vi "UHR-Fleezers Control (host) - 12.1.vi"() -> ()   [LabVIEW 2012] (continued)
  in  "Limits Enable":bool=TRUE caption="Enable"
  out "AI labels":string[](array[string])=["T1 Y", "T1 X", "T1 Sum", "T2 Y", "T2 X", "T2 Sum", "T1 FB X", "T1 FB Sum", "T2 FB X", "T2 FB Sum", "PSD Y", "PSD X", "PSD Y Sum"]
  in  "Save Trap Pos. Data":bool=TRUE
  in  "Lower Ch. Cap.":bool
  in  "Top 3 Harvard Syringe Pump Serial Port":refnum<visa-resource-name>="Top3Harvard"
  # "After"
  # "During"
  # "Trap On?"
  # "BD Flow ON?"
  # "Samp Flow ON?"
  # "Trap Trig. Fl.?"
  # "Zero It"
  # "Floor it\n(e.g., hp unwinding)"
  # "1"
  # "2"
  # "Fl. Down"
  # "Fl. Up"
  # "Bead sep"
  # "Trap Display:"
  # "APD Display:"
  # "DAQ"
  # "Trap Manipulation"
  # "Data Saving"
  # "Bead Calibration"
  # "Bottom Pump (#1)"
  # "Central Sample Channels"
  # "Top Pump (#3)"
  # "Rate param is ul/h\nVolume param is ul"
  # "Chemyx Pump 2"
  # "Units: \n1 = ml/m\n2 = ml/h\n3 = ul/m\n4 = ul/h"
  # "X"
  # "Amp switch 1st is disabled in the fpga"
  # "Y"
  # "Oscillate Set 1 freq. (debugging)"
  # "BD 1"
  # "BD 2"
  # "AOD Raster Scan"
  # "Approx. trap separations"
  # "X"
  # "Y"
  # "FPGA\nreading"
  # "DMA\ntransfer"
  # "APD Gates"
  # "APD 2"
  # "APD 1"
  # "X"
  # "2D"
  # "Y"
  # "1D"
  # "Green Laser Interlacing"
  # "Green FB Measurement"
  # "Digital Gate"
  # "Current Analog Control"
  # "Total AI Rates (NOT rates/trap)"
  # "(Samples/trap x Trap Sets)"
  # "(Samples/channel x\n8 if averaging (8 channels)\n4 if no averaging)"
  # "Trap 1"
  # "Trap 2"
  # "Flour./Trap 3"
  # "External Video Window"
  # "MCL Position Debugging"
  # "Temporary Control Storage\n(these used to be somewhere else, still want to keep them)"
  # "Y"
  # "X"
  # "Trap Position Difference Limits"
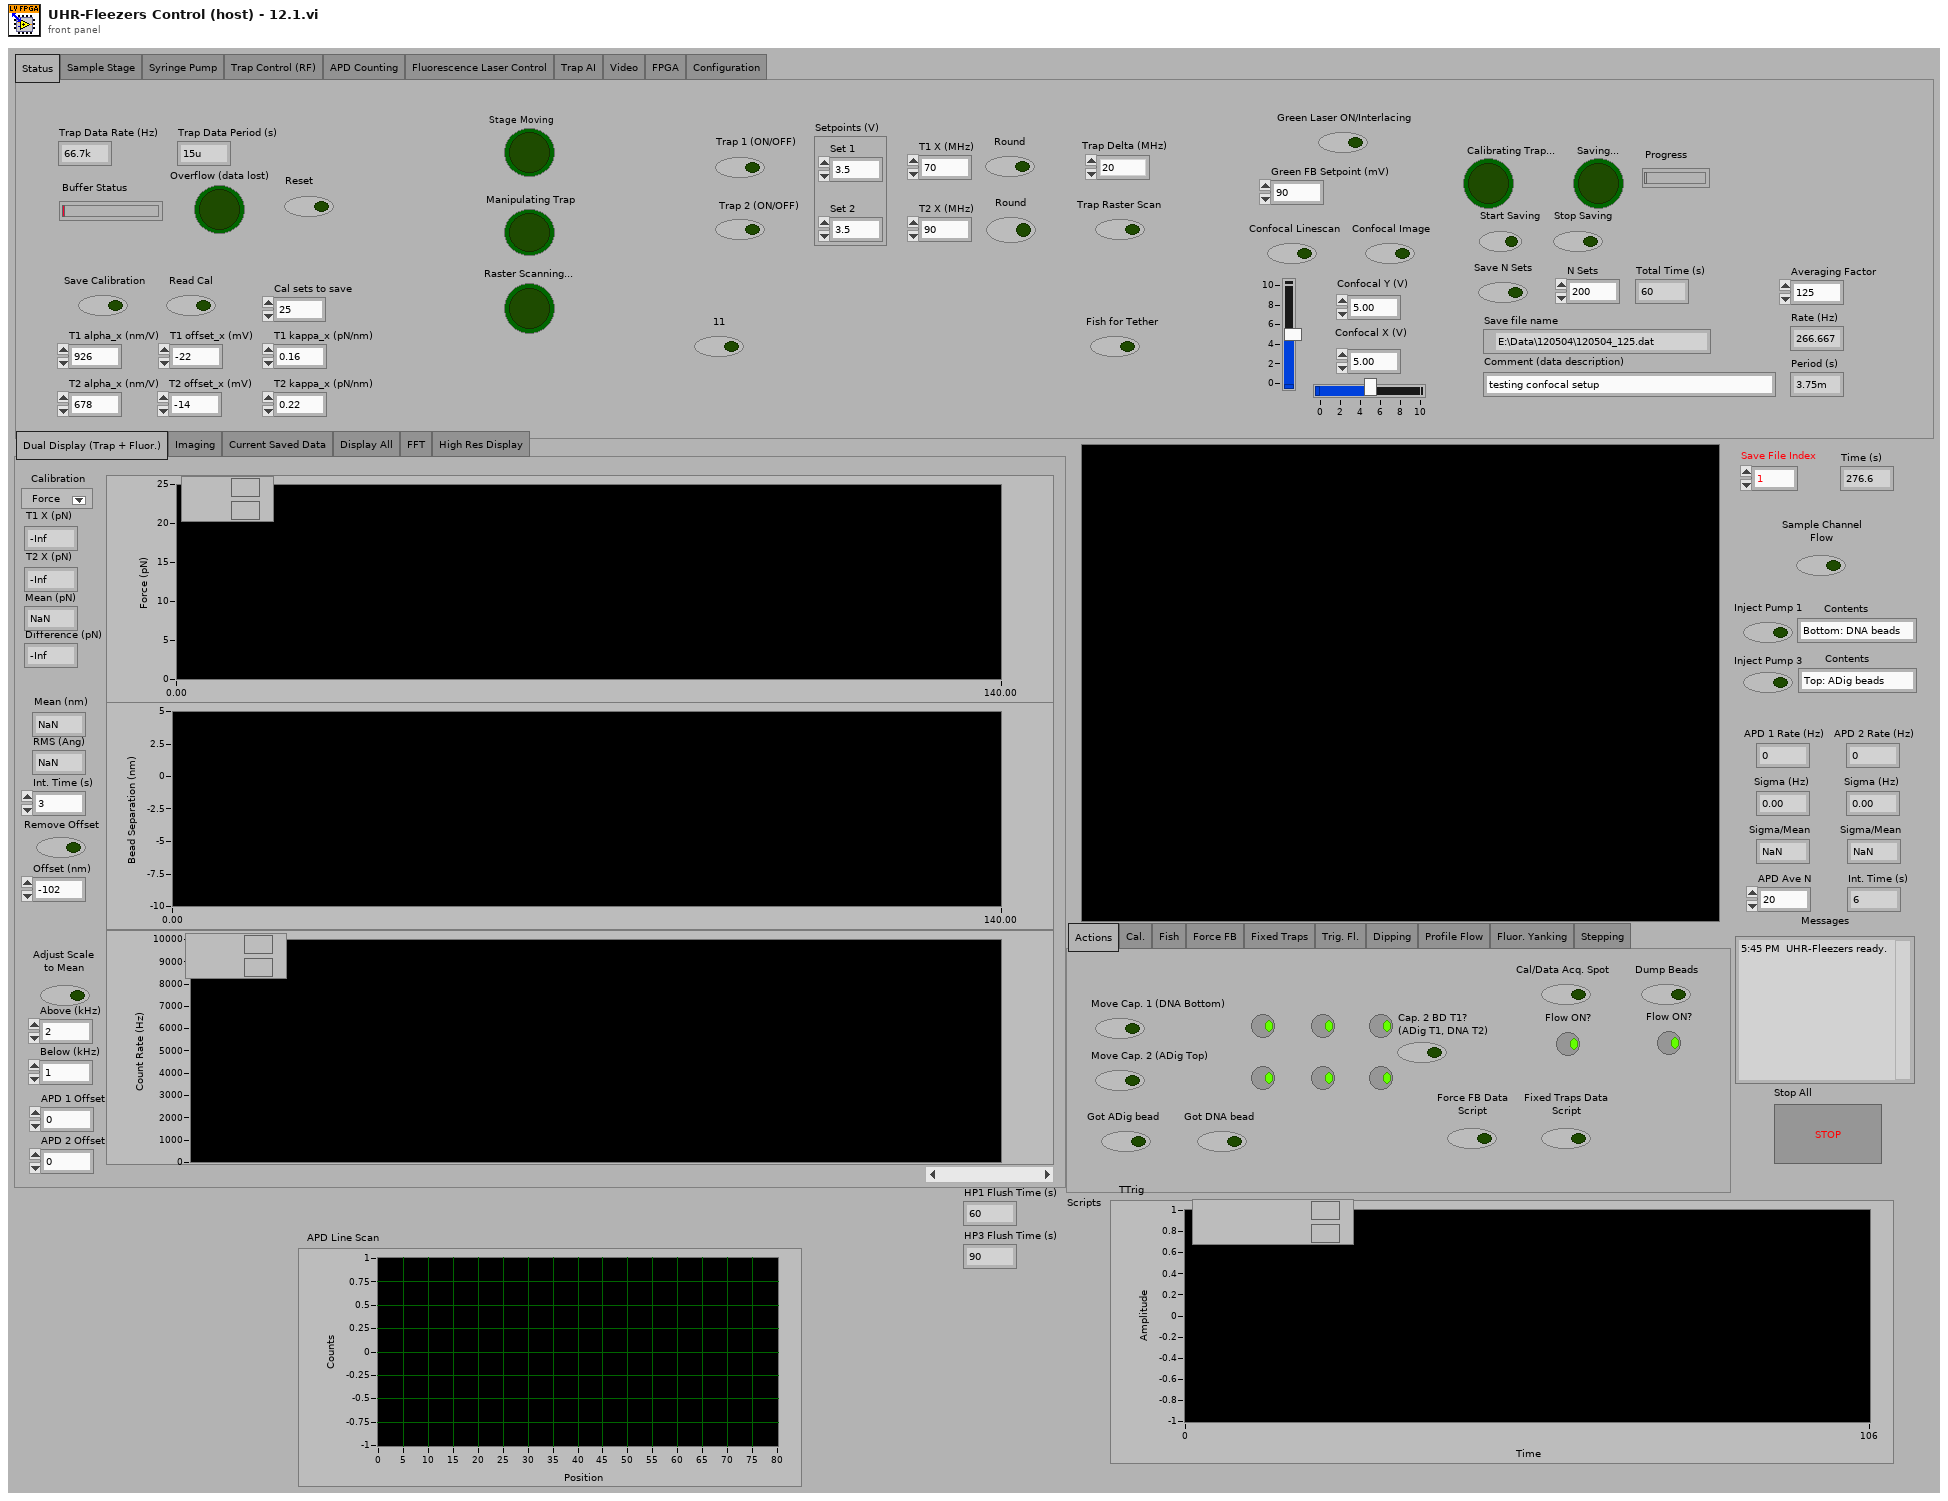
[diagram p1: front panel]
types:
  T1 = enum32{"Actions", "Cal.", "Fish", "Force FB", "Fixed Traps", "Trig. Fl.", "Dipping", "Profile Flow", "Fluor. Yanking", "Stepping"}
  T2 = typedef "IMAQ Image.ctl" = refnum<image>
  T3 = enum32{"Dual Display (Trap + Fluor.)", "Imaging", "Current Saved Data", "Display All", "FFT", "High Res Display"}
  T4 = enum32{"Status", "Sample Stage", "Syringe Pump", "Trap Control (RF)", "APD Counting", "Fluorescence Laser Control", "Trap AI", "Video", "FPGA", "Configuration"}
  T5 = cluster{"Pump 1":cluster{"Diameter (mm)":dbl, "Units":dbl, "Volume":dbl, "Rate":dbl}, "Pump 2":cluster{"Diameter (mm)":dbl, "Units":dbl, "Volume":dbl, "Rate":dbl}, "Pump 3":cluster{"Diameter (mm)":dbl, "Units":dbl, "Volume":dbl, "Rate":dbl}}
  T6 = enum32{"IR Laser Interlacing (Direct RF Board Control Method)", "AOD Raster Scan", "Feedback on Trap Intensity", "Feedback on Trap Position"}
  T7 = typedef "LVPoint32TypeDef.ctl" = cluster{"Horizontal":i32, "Vertical":i32}
  T8 = cluster{"Scan Range AOD (nm) 2":dbl, "Step Size AOD (nm) 2":dbl, "Scan Speed AOD (nm/s) 2":dbl, "Number of scans (AOD) 2":u16, "Label":string}[]
  T9 = cluster{"proportional gain (Kc)":i16, "integral gain (Kc*Ts/Ti)":i16, "derivative gain (Kc*Td/Ts)":i16}
  T10 = cluster{"Trap 1":fxp<+/-,16,1>, "Trap 2":fxp<+/-,16,1>}
  T11 = cluster{"proportional gain (Kc)":fxp<+/-,16,8>, "integral gain (Kc*Ts/Ti)":fxp<+/-,16,8>, "derivative gain (Kc*Td/Ts)":fxp<+/-,16,8>}
  T12 = cluster{"output high":fxp<+/-,16,1>, "output low":fxp<+/-,16,1>}
  T13 = cluster{"Set 1":fxp<+/-,16,1>, "Set 2":fxp<+/-,16,1>}
  T14 = cluster{"Set 1":bool, "Set 2":bool, "Set 3":bool}
  T15 = typedef "LVMinMaxIncTypeDef.ctl" = cluster{"Minimum":dbl, "Maximum":dbl, "Increment":dbl}
  T16 = typedef "Image Type" = u32
  T17 = typedef "nirio_resource_hc.ctl" = tag
  T18 = typedef "openfpgaref.8.6.ctl" = refnum<k20>
  T19 = cluster{"New Image":T2, "New Image":T2, "New Image":T2, "New Image":T2}
  T20 = typedef "XDNodeRunTimeDep.lvlib/timing_clust.ctl" = cluster{"Expected End [f-1]":u64, "Actual End [f-1]":u64, "Finished Late? [f-1]":bool, "Expected End [i-1]":u64, "Actual End [i-1]":u64, "Finished Late? [i-1]":bool, "Expected Start [i]":u64, "Actual Start [i]":u64, "Expected Start [f]":u64, "Actual Start [f]":u64, "Source Name":string, "Structure Name":string, "Period":i64, "Deadline":i64, "Offset":i64, "Start":i64, "Priority":i32, "Timeout":i32, "Mode":T21, "Wakeup Reason":T22, "Error":errorcluster, "Source Type":string, "Secondary Source Type":string, "Global End Time":u64, "Global Start Time":u64, "Frame Duration":u64, "Iteration Duration":u64, "Assigned CPU":i32, "I/O Scan Engine Mode":u32}
  T21 = typedef "XDNodeRunTimeDep.lvlib/nitl_modes.ctl" = enum32{"No Change", "Process missed periods, maintain original phase", "Discard missed periods, maintain original phase", "Process missed periods, ignore original phase", "Discard missed periods, ignore original phase"}
  T22 = typedef "XDNodeRunTimeDep.lvlib/wakeup.ctl" = enum32{"Normal", "Aborted", "Asynchronous wakeup", "Timing source error", "Timed loop error", "Timeout"}
  T23 = cluster{"Left":i32, "Top":i32, "Width":u32, "Height":u32}
  T24 = cluster{cluster{"Left":i32, "Top":i32, "Width":u32, "Height":u32}}[]
  T25 = enum32{"setting", "request", "request control", "info", "statistics", "system settings", "I/O sub system", "HRT control", "camera descriptions", "device specific data", "event sub system settings", "event sub system results", "image memory manager"}
  T26 = typedef "AviRefnum.ctl" = refnum<k1>
  T27 = typedef "imagedata.ctl" = cluster{"image type":i32, "image depth":i32, "image":u8[], "mask":u8[], "colors":u32[], "Rectangle":cluster{"left":i16, "top":i16, "right":i16, "bottom":i16}}
  T28 = enum32{"Normal Display", "Dual Display (APD)", "FFT", "High Res Display"}
  T29 = cluster{"Origin Pixel":cluster{"X":sgl, "Y":sgl}, "Angle Relative to Horizontal (deg)":sgl, "Axis Reference":u32}
  T30 = typedef "Simple Grid Descriptor" = cluster{"X Step":sgl, "Y Step":sgl, "Unit":T31}
  T31 = typedef "Image Unit" = enum32{"Undefined", "Angström", "Micrometer", "Millimeter", "Centimeter", "Meter", "Kilometer", "Microinch", "Inch", "Feet", "Nautical miles", "Standard miles", "Steps"}
  T32 = cluster{"averaging mode":u16, "weighting mode":u16, "number of averages":u32}
  T33 = cluster{"dB On (F)":bool, "unwrap phase (F)":bool, "convert to degree (F)":bool}
  T34 = enum16{"open", "replace", "create", "open or create", "replace or create", "replace or create with confirmation"}
  T35 = enum16{"big-endian, network order", "native, host order", "little-endian"}
  T36 = cluster{string, string, string, string, string, string, string, string}
  T37 = cluster{string, string, string, string, string, string, string, string, string, string, string, string}
  T38 = cluster{string, string, string, string, string, string, string, string, string, string, string, string, string}
  T39 = cluster{string, string, string, string, string, string, string, string, string, string, string, string, string, string}
  T40 = cluster{"BD 1 Frequency 1 (MHz)":dbl, "BD 1 Frequency 2 (MHz)":dbl}
  T41 = cluster{"f0":dbl, "df":dbl, "magnitude":dbl[]}[][]
  T42 = cluster{"Scan Range AOD (nm) 2":dbl, "Step Size AOD (nm) 2":dbl, "Scan Speed AOD (nm/s) 2":dbl, "Number of scans (AOD) 2":u16, "Label":string}
  T43 = cluster{"[0]":dbl, "[1]":dbl, "[2]":dbl, "[3]":dbl, "[4]":dbl, "[5]":dbl}
  T44 = cluster{"Diameter (mm)":dbl, "Units":dbl, "Volume":dbl, "Rate":dbl}
diagram:
  w34 = u16 20 items=["1.0"=10, "1.5"=15, "2.0"=20] ("stop bits (10: 1 bit)")
  w37 = u16 20 items=["1.0"=10, "1.5"=15, "2.0"=20] ("stop bits (10: 1 bit)")
  w91 = u16 20 items=["1.0"=10, "1.5"=15, "2.0"=20] ("stop bits (10: 1 bit)")
  w98 = T16 2 items=["Grayscale (U8)", "Grayscale (I16)", "Grayscale (SGL)", "Complex (CSG)", "RGB (U32)", "HSL (U32)", "RGB (U64)", "Grayscale (U16)"] ("Image Type")
  w227 = 10.0 ("y")
  w226 = 32767.0 ("y")
  w242 = 6.0  # clock mult.
  w243 = 49152000.0  # TCXO frequ.
  # "Bottom 1 Harvard"
  # "Top 3 Harvard"
  # "Center Harvard"
  # "Bottom 1 Harvard"
  # "Top 3 Harvard"
  # "Center Harvard"
  n1 = Build Array("DIO count 1 (ticks)", "DIO count 2 (ticks)", "DIO count 3 (ticks)") -> (w147:u32[])
  n2 = local read "AO1"() -> (w221:dbl)
  n3 = local read "AO2"() -> (w220:dbl)
  n4 = local read "Scan Increment (MHz)"() -> (w238:dbl)
  n5 = local read "Continuous MCL Scanning"() -> (w208:bool)
  n6 = local read "Fast Scan Dir"() -> (w207:bool)
  n7 = local read "Number of scans (MCL)"() -> (w209:u64)
  n8 = property on="AI Count (ticks)" class="DigNum (strict)"("Val(Sgnl)"="AI Count (ticks)") -> ()  [unwired: 2 in, 2 out]
  n9 = Multiply(x=w221, y=w226) -> (x*y=w223:dbl)
  n10 = Multiply(x=w220, y=w226) -> (x*y=w225:dbl)
  n11 = Divide(x=w223, y=w227) -> (x/y=w222:dbl)
  n12 = Divide(x=w225, y=w227) -> (x/y=w224:dbl)
  n13 = To Word Integer(number=w222) -> (16bit integer=w219:i16)
  n14 = To Word Integer(number=w224) -> (16bit integer=w218:i16)
  n15 = Not(x=w207) -> (.not. x?=w202:bool)
  n16 = local read "Cycles/step (MCL)"() -> (w210:u64)
  n17 = Multiply(x=w238, y=1000.0) -> (x*y=w245:dbl)
  n18 = local read "Scan steps (MCL)"() -> (w211:u64)
  n19 = local write "Trap Pos FIFO Timeout"(u16 0 ("Trap Pos FIFO Timeout")) -> ()
  n20 = local read "Desired Scan Incr (V)"() -> (w213:dbl)
  n21 = Scale By Power Of 2(n=48, x=w245) -> (x*2^n=w246:dbl)
  n22 = Unbundle By Name(cluster{"output high":i16, "output low":i16} {"output high"=3000, "output low"=0} ("FB output range 1")) -> ("output high"=w14:i16, "output low"=w13:i16)
  n23 = Multiply(x=w243, y=w242) -> (x*y=w241:dbl)
  n24 = Divide(x=w246, y=w241) -> (x/y=w240:dbl)
  n25 = local read "Setpoints (V)"() -> (w257:cluster{"Set 1":dbl, "Set 2":dbl})
  n26 = To Quad Integer(1:w240) -> (0:w237:i64)
  n27 = Divide(x=40000000.0, y="AI Count (ticks)") -> (x/y=w198:dbl)
  n28 = Multiply(x=w213, y=32767.0) -> (x*y=w215:dbl)
  n29 = local read "Trap Intensity PID Gains"() -> (w252:T9)
  n30 = local read "Number Interlace Sets"() -> (w140:u8)
  n31 = Split 1D Array(array=w147, index=w140) -> (first subarray=w149:u32[])  [unwired: 1 out]
  n32 = Add Array Elements(numeric array=w149) -> (sum=w148:u32)
  n33 = local read "# Samples/channel"() -> (w230:u32)
  n34 = local read "Number of F/B Scans (AOD)"() -> (w231:u16)
  n35 = local read "Not-Interlacing Set"() -> (w139:enum32{"Set 1", "Set 2", "Set 3"})
  n36 = To Unsigned Byte Integer(number=w139) -> (unsigned 8bit integer=w145:u8)
  n37 = Index Array(array=w147, index=w145) -> (element=w146:u32)
  n38 = local read "Feedback On/Off"() -> (w260:cluster{"Set 1":bool, "Set 2":bool})
  n39 = local read "Scan steps (AOD)"() -> (w236:u64)
  n40 = local read "All FB On/Off"() -> (w261:bool)
  n41 = local read "Cycles/step (AOD)"() -> (w235:u64)
  n42 = local write "AI rate (Hz)"(w198) -> ()
  n43 = Divide(x=w215, y=10.0) -> (x/y=w214:dbl)
  n44 = Multiply(x=w236, y=w235) -> (x*y=w234:u64)
  n45 = Unbundle By Name(w252) -> ("proportional gain (Kc)"=w18:i16, "integral gain (Kc*Ts/Ti)"=w17:i16, "derivative gain (Kc*Td/Ts)"=w16:i16)
  n46 = Multiply(x=3276.7, y=w257) -> (x*y=w256:cluster{"Set 1":dbl, "Set 2":dbl})
  n47 = xnode "Open FPGA VI Reference"("resource name"=T17 "750kHzDAQ") -> ("FPGA VI Reference Out"=w251:T18, "error out"=w250:errorcluster)  [unwired: 1 in]
  n48 = To Word Integer(number=w214) -> (16bit integer=w212:i16)
  n49 = Multiply(x=w234, y=u64 2) -> (x*y=w232:u64)
  n50 = Divide(x=w198, y="FPGA Ave.") -> (x/y=w199:dbl)
  n51 = To Word Integer(number=w256) -> (16bit integer=w255:cluster{"Set 1":i16, "Set 2":i16})
  n52 = Multiply(x=w232, y=w231) -> (x*y=w229:u64)
  n53 = local read "Sets to FIFO (Traps)"() -> (w22:T14)
  n54 = local write "Ave. Rate (Hz)"(w199) -> ()
  n55 = Divide(x=w229, y=w230) -> (x/y=w228:dbl)
  n56 = Unbundle By Name(w255) -> ("Set 1"=w254:i16, "Set 2"=w253:i16)
  n57 = local read "2D or 1D Scan"() -> (w159:bool)
  n58 = local write "Data points/scans"(w229) -> ()
  n59 = local read "Scan BD"() -> (w247:bool)
  n60 = And(x=w260, y=w261) -> (x .and. y?=w259:cluster{"Set 1":bool, "Set 2":bool})
  n61 = local write "Data points/scan (f/b)"(w232) -> ()
  n62 = Reciprocal(x=w199) -> (1/x=w200:dbl)
  n63 = local read "N Acq Sets (Traps + Fl.)"() -> (w191:i16)
  n64 = local write "N sets should be saved"(w228) -> ()
  n65 = xnode "Invoke Method"("FPGA VI Reference In"=w251, "error in"=w250) -> ("FPGA VI Reference Out"=w158:T18, "error out"=w167:errorcluster)
  n66 = Unbundle By Name(w259) -> ("Set 1"=w263:bool, "Set 2"=w262:bool)
  n67 = local read "Interlace"() -> (w141:bool)
  n68 = Select(t=w148, s=w141, f=w146) -> (s? t:f=w138:u32)
  n69 = local write "Update Count (MCL)"(w138) -> ()
  n70 = local write "Total Counts (ticks)"(w138) -> ()
  n71 = local write "Ave. Period (s)"(w200) -> ()
  n72 = Unbundle By Name(w22) -> ("Set 1"=w21:bool, "Set 2"=w20:bool, "Set 3"=w19:bool)
  n73 = property on="2D or 1D Scan" class="Bool (strict)"("Val(Sgnl)"=w159) -> ()  [unwired: 2 in, 2 out]
  n74 = local read "GI Frequency, OFF count"() -> (w65:u32)
  n75 = local read "GI Frequency, ON count"() -> (w56:u32)
  n76 = local read "APD Gate OFF Count"() -> (w62:u32)
  n77 = local read "APD Gate ON Count"() -> (w58:u32)
  n78 = xnode "Read/Write Control"("FPGA VI Reference In"=w157, "error in"=w167, "ai count"="AI Count (ticks)", "Interlace ON/OFF"=w141, "Number Interlace Cycles"=w140, "Set 1"=w21, "Set 2"=w20, "Set 3"=w19, "FB On/Off Set 1"=w263, "FB On/Off Set 2"=w262, "Interlace Off Parameters"=w139, "FB Setpoint Set 1"=w254, "FB Setpoint Set 2"=w253, "P1"=w18, "I1"=w17, "D1"=w16, "FB1 output high"=w14, "FB1 output low"=w13, "Cycles per step"=w235, "Scan BD"=w247, "Number of scans"=w231, "Scan steps"=w236, "Scan freq.  increment"=w237, "AO1"=w219, "AO2"=w218, "Scan freq.  increment (MCL)"=w212, "Scan steps (MCL)"=w211, "Cycles per step (MCL)"=w210, "Number of scans (MCL)"=w209, "MCL count"=w138, "Cont. Scan (MCL)"=w208, "MCL Scan Axis"=w202, "1D or 2D Scan?"=w159, "N of AI1 Int Acq Sets"=w191, "Amp switch delay"="Amp switch delay", "Swap F1 and F2"="Swap F1 and F2", "APD to FIFO"=FALSE, "DIO count 1 (ticks)"="DIO count 1 (ticks)", "DIO count 2 (ticks)"="DIO count 2 (ticks)", "DIO count 3 (ticks)"="DIO count 3 (ticks)") -> ("FPGA VI Reference Out"=w69:T18, "error out"=w67:errorcluster)  [unwired: 1 in]
  n79 = local read "On one out of X cycles"() -> (w64:u32)
  n80 = local read "APD Integration Time (s)"() -> (w48:dbl)
  n81 = local read "DMA Update Period (s)"() -> (w47:dbl)
  n82 = Add(x=w58, y=w62) -> (x+y=w60:u32)
  n83 = Add(x=w56, y=w65) -> (x+y=w63:u32)
  n84 = local read "Green Laser ON/Interlacing"() -> (w136:bool)
  n85 = local read "Green laser mode"() -> (w137:enum32{"Laser ON", "Laser OFF", "Interlace"})
  n86 = local read "Trap Pos. FB Range"() -> (w12:T12)
  n87 = local read "Trap Pos. FB Gains"() -> (w11:T11)
  n88 = Multiply(x=w60, y=w64) -> (x*y=w61:u32)
  n89 = Multiply(x=w64, y=w63) -> (x*y=w55:u32)
  n90 = Reciprocal(x=w48) -> (1/x=w45:dbl)
  n91 = Multiply(x=w48, y=40000000.0) -> (x*y=w44:dbl)
  n92 = Divide(x=w47, y=w48) -> (x/y=w50:dbl)
  n93 = Multiply(x="Current When FB OFF (%)", y=655.35) -> (x*y=w125:dbl)
  n94 = local read "Trap Pos. AI1 X Pre-scale"() -> (w79:u16)
  n95 = local read "Invert APD Gate"() -> (w54:bool)
  n96 = Multiply(x="Green FB Setpoint (mV)", y=3.2767) -> (x*y=w122:dbl)
  n97 = local read "APD Gate"() -> (w53:enum32{"ON", "OFF", "Interlace"})
  n98 = local read "Trap Pos FB Int Count"() -> (w73:u16)
  n99 = Subtract(x=w61, y=w58) -> (x-y=w59:u32)
  n100 = local write "Green FB Count"(w55) -> ()
  n101 = local write "APD Acq Rate (Hz)"(w45) -> ()
  n102 = local read "Differential FB?"() -> (w39:bool)
  n103 = To Unsigned Long Integer(number=w44) -> (unsigned 32bit integer=w42:u32)
  n104 = local read "Neg. TTrig FPGA"() -> (w41:bool)
  n105 = Multiply(x=2.0, y=w50) -> (x*y=w49:dbl)
  n106 = local read "Invert GI"() -> (w133:bool)
  n107 = To Unsigned Word Integer(number=w125) -> (unsigned 16bit integer=w123:u16)
  n108 = Subtract(x=w55, y=w56) -> (x-y=w57:u32)
  n109 = local write "APD Samples/FIFO Acq."(w50) -> ()
  n110 = To Word Integer(number=w122) -> (16bit integer=w120:i16)
  n111 = Unbundle By Name("Green FB Gains") -> ("proportional gain (Kc)"=w3:i16, "integral gain (Kc*Ts/Ti)"=w2:i16, "derivative gain (Kc*Td/Ts)"=w1:i16)
  n112 = local write "APD Elements/DMA read"(w49) -> ()
  n113 = case shown="False" w136 {
    tunnel: w137 -> [_ w289]
    tunnel: [enum32{"Laser ON", "Laser OFF", "Interlace"}."Laser OFF" ("Green laser mode") w289] -> w132
    frame False {
    }
    frame True {
    }
  }
  n114 = local write "APD Int. Count"(w42) -> ()
  n115 = Unbundle By Name(w11) -> ("proportional gain (Kc)"=w7:fxp<+/-,16,8>, "integral gain (Kc*Ts/Ti)"=w6:fxp<+/-,16,8>, "derivative gain (Kc*Td/Ts)"=w5:fxp<+/-,16,8>)
  n116 = Unbundle By Name(w12) -> ("output high"=w10:fxp<+/-,16,1>, "output low"=w8:fxp<+/-,16,1>)
  n117 = local read "Trap Pos FB Monitor\nT1 or T2"() -> (w84:bool)
  n118 = local read "APD 1 AO Mult."() -> (w52:i16)
  n119 = local read "Trap Pos FB Negate Action"() -> (w83:bool)
  n120 = local read "APD 2 AO Mult."() -> (w51:i16)
  n121 = local read "Trap Pos. FB Offset Factor"() -> (w82:i64)
  n122 = local read "Trap Pos. FB Mult Factor"() -> (w81:i64)
  n123 = xnode "Read/Write Control"("FPGA VI Reference In"=w69, "error in"=w67, "Invert APD Gate"=w54, "APD Gate ON Count"=w58, "APD Gate OFF Count"=w59, "APD Acq Rate Count"=w42, "APD Gate Operating Mode"=w53, "APD 1 AO scale factor"=w52, "APD 2 AO scale factor"=w51, "Green interlace ON count"=w56, "Green interlace OFF count"=w57, "Green interlace ON count 2"=w56, "Green interlace OFF count 2"=w57, "Green FB Count"=w55) -> ("FPGA VI Reference Out"=w68:T18, "error out"=w66:errorcluster)
  n124 = xnode "Read/Write Control"("FPGA VI Reference In"=w68, "error in"=w66, "Invert GI 2"=w133, "Operating Mode 2"=w132, "P3"=w3, "I3"=w2, "D3"=w1, "Green FB Setpoint"=w120, "Green FB On/Off"="Green FB On/Off", "Current Out"=w123, "Green int current ON count adj"="Green int current ON count adj", "Operating Mode"=w132, "Invert GI"=w133, "Trap Pos FB Monitor T1 or T2"=w84, "Trap Pos FB Negate Action"=w83, "Trap Pos. FB Offset Factor"=w82, "Trap Pos. FB Mult Factor"=w81, "Force feedback"=FALSE, "AI1 X Scale"=w79, "Trap Pos to FIFO"=TRUE, "Trap Pos FB Int Count"=w73, "TTrig Negate Pos"=w41, "FB Trig Integrate"="FB Trig Integrate", "Diff FB Measurement?"=w39, "Negate Diff?"="Negate Diff?", "P2"=w7, "I2"=w6, "D2"=w5, "FB2 output high"=w10, "FB2 output low"=w8) -> ("FPGA VI Reference Out"=w134:T18, "error out"=w135:errorcluster)
  n125 = xnode "Invoke Method"("FPGA VI Reference In"=w134, "error in"=w135, "Requested Depth"="Trap AI FIFO Depth") -> ("FPGA VI Reference Out"=w87:T18, "error out"=w86:errorcluster)  [unwired: 1 out]
  n126 = xnode "Invoke Method"("FPGA VI Reference In"=w87, "error in"=w86, "Requested Depth"="Trap Position FIFO Depth") -> ("FPGA VI Reference Out"=w75:T18, "error out"=w74:errorcluster)  [unwired: 1 out]
  n127 = flat-sequence {
    tunnel: w158 -> [w294]
    tunnel: [w294] -> w157
    tunnel: [w293] -> w156
    tunnel: [w292] -> w155
    tunnel: [w290] -> w153
    tunnel: [w291] -> w154
    frame #0 {
      w291 = T15 {"Minimum"=0.0, "Maximum"=40.0, "Increment"=1.0} ("Min Max Inc")
      w290 = T15 {"Minimum"=0.0, "Maximum"=50.0, "Increment"=1.0} ("Data Entry Limits")
      w293 = T15 {"Minimum"=60.0, "Maximum"=90.0, "Increment"=1.0} ("Min Max Inc")
      w292 = T15 {"Minimum"=0.0, "Maximum"=50.0, "Increment"=1.0} ("Data Entry Limits")
      n128 = property on="BD 2 Frequency 1 (MHz)" class="DigNum (strict)"("Data Range"=w291) -> ()  [unwired: 2 in, 2 out]
      n129 = property on="BD 2 Frequency 3 (MHz)" class="DigNum (strict)"("Data Range"=w291) -> ()  [unwired: 2 in, 2 out]
      n130 = property on="BD 2 Frequency 2 (MHz)" class="DigNum (strict)"("Data Range"=w291) -> ()  [unwired: 2 in, 2 out]
      n131 = property on="BD 1 Frequency 1 (MHz)" class="DigNum (strict)"("Data Range"=w293) -> ()  [unwired: 2 in, 2 out]
      n132 = property on="BD 1 Frequency 2 (MHz)" class="DigNum (strict)"("Data Range"=w293) -> ()  [unwired: 2 in, 2 out]
      n133 = property on="BD 1 Frequency 3 (MHz)" class="DigNum (strict)"("Data Range"=w293) -> ()  [unwired: 2 in, 2 out]
      n134 = property on="BD 2 Amplitude 1 (%)" class="DigNum (strict)"("Data Range"=w290) -> ()  [unwired: 2 in, 2 out]
      n135 = property on="BD 2 Amplitude 2 (%)" class="DigNum (strict)"("Data Range"=w290) -> ()  [unwired: 2 in, 2 out]
      n136 = property on="BD 2 Amplitude 3 (%)" class="DigNum (strict)"("Data Range"=w290) -> ()  [unwired: 2 in, 2 out]
      n137 = property on="BD 1 Amplitude 3 (%)" class="DigNum (strict)"("Data Range"=w292) -> ()  [unwired: 2 in, 2 out]
      n138 = property on="BD 1 Amplitude 2 (%)" class="DigNum (strict)"("Data Range"=w292) -> ()  [unwired: 2 in, 2 out]
      n139 = property on="BD 1 Amplitude 1 (%)" class="DigNum (strict)"("Data Range"=w292) -> ()  [unwired: 2 in, 2 out]
      "X RF Frequency Limits (MHz)" <- w293
      "X RF Amplitude Limits (%)" <- w292
      "Y RF Amplitude Limits (%)" <- w290
      "Y RF Frequency Limits (MHz)" <- w291
    }
  }
  n140 = xnode "Invoke Method"("FPGA VI Reference In"=w75, "error in"=w74) -> ("FPGA VI Reference Out"=w166:T18, "error out"=w165:errorcluster)  [unwired: 1 in]
  n141 = flat-sequence "Initial FPGA Loop Relative Phase Adjustment" {
    tunnel: "Initial Phase Adjustment (AI1)" -> [w305]
    tunnel: "Initial Phase Adjustment (GI)" -> [w304]
    tunnel: w166 -> [w303]
    tunnel: w165 -> [w302]
    tunnel: "Initial Phase Adj. (MCL)" -> [w301]
    tunnel: [w306] -> w175
    tunnel: [w300] -> w171
    tunnel: "Initial Phase Adjustment (APD Acq)" -> [w299]
    tunnel: "Initial Phase Adjustment (APD 1 Gate)" -> [w298]
    tunnel: "Initial Phase Adjustment (Green FB)" -> [w297]
    tunnel: "Initial Phase Adjustment (GI) 2" -> [w296]
    tunnel: "Initial Phase Adjustment (APD 2 Gate)" -> [w295]
    tunnel: w175 -> [w308]
    tunnel: [w309] -> w172
    tunnel: w171 -> [w309]
    tunnel: [w308] -> w170
    tunnel: w172 -> [w312]
    tunnel: w170 -> [w311]
    tunnel: [w314] -> w169
    tunnel: [w313] -> w168
    tunnel: [w316] -> w173
    tunnel: [w317] -> w174
    tunnel: w169 -> [w317]
    tunnel: w168 -> [w316]
    frame #0 {
      n142 = xnode "Read/Write Control"("FPGA VI Reference In"=w303, "error in"=w302, "Phase count adjustment"=w305, "Phase count adjustment (GI)"=w304, "Phase count adjustment (MCL)"=w301, "Phase Count Adjustment (APD Acq)"=w299, "Phase count adjustment (APD 1 Gate)"=w298, "Phase count adjustment (APD 2 Gate)"=w295, "Phase count adjustment (Green FB)"=w297, "Phase count adjustment (GI) 2"=w296) -> ("FPGA VI Reference Out"=w300:T18, "error out"=w306:errorcluster)
    }
    frame #1 {
      n143 = Wait (ms)(milliseconds to wait=u32 100) -> ()  [unwired: 1 out]
    }
    frame #2 {
      w310 = TRUE
      n144 = xnode "Read/Write Control"("FPGA VI Reference In"=w312, "error in"=w311, "+ phase"=w310, "+ phase (GI)"=w310, "+ phase (MCL)"=w310, "+ phase (APD Acq)"=w310, "+ phase (APD 1 Gate)"=w310, "+ phase (APD 2 Gate)"=w310, "+ phase (Green FB)"=w310, "+ phase (GI) 2"=w310) -> ("FPGA VI Reference Out"=w313:T18, "error out"=w314:errorcluster)
    }
    frame #3 {
      n145 = Wait (ms)(milliseconds to wait=u32 100) -> ()  [unwired: 1 out]
    }
  }
  n146 = local read "Phase adj. (Green FB)"() -> (w150:i16)
  n147 = local read "Phase adj. (GI) 2"() -> (w126:i16)
  n148 = local read "Phase adjust (MCL)"() -> (w203:i16)
  n149 = local read "Phase adj. (AI1)"() -> (w205:i16)
  n150 = local read "Phase adj. (GI)"() -> (w204:i16)
  n151 = xnode "Read/Write Control"("FPGA VI Reference In"=w173, "error in"=w174, "Phase count adjustment"=w205, "Phase count adjustment (GI)"=w204, "Phase count adjustment (MCL)"=w203, "Phase Count Adjustment (APD Acq)"="Phase Adj. (APD Acq)", "Phase count adjustment (APD 1 Gate)"="Phase Adj. (APD 1 Gate)", "Phase count adjustment (APD 2 Gate)"="Phase Adj. (APD 2 Gate)", "Phase count adjustment (Green FB)"=w150, "Phase count adjustment (GI) 2"=w126) -> ("FPGA VI Reference Out"=w112:T18, "error out"=w180:errorcluster)
  n152 = call "Initialize RF boards - interlace 3.vi"("error in"=w180, "FPGA VI Reference In"=w112) -> ("error out"=w178:errorcluster, "FPGA VI Reference Out"=w179:T18)
  n153 = call "set RF board frequency - interlace.vi"("Board 2 Frequency Limits"=w154, "Board 1 Frequency Limits"=w156, "error in"=w178, "FPGA VI Reference In"=w179, "Board 2 Frequency 3 (MHz)"="BD 2 Frequency 3 (MHz)", "Board 1 Frequency 3 (MHz)"="BD 1 Frequency 3 (MHz)", "Board 2 Frequency 2 (MHz)"="BD 2 Frequency 2 (MHz)", "Board 2 Frequency 1 (MHz)"="BD 2 Frequency 1 (MHz)", "Board 1 Frequency 2 (MHz)"="BD 1 Frequency 2 (MHz)", "Board 1 Frequency 1  (MHz)"="BD 1 Frequency 1 (MHz)") -> ("error out"=w278:errorcluster, "FPGA VI Reference Out"=w279:T18)
  n154 = call "set RF board amplitude - interlace.vi"("Board 2 Amplitude Limits"=w153, "Board 1 Amplitude Limits"=w155, "error in"=w278, "FPGA VI Reference In"=w279, "Board 2 Amplitude 3 (%)"="BD 2 Amplitude 3 (%)", "Board 1 Amplitude 3 (%)"="BD 1 Amplitude 3 (%)", "Board 2 Amplitude 2 (%)"="BD 2 Amplitude 2 (%)", "Board 2 Amplitude 1 (%)"="BD 2 Amplitude 1 (%)", "Board 1 Amplitude 2 (%)"="BD 1 Amplitude 2 (%)", "Board 1 Amplitude 1 (%)"="BD 1 Amplitude 1 (%)") -> ("error out"=w266:errorcluster, "FPGA VI Reference Out"=w267:T18)
  n155 = flat-sequence {
    tunnel: w267 -> [w327]
    tunnel: w266 -> [w326]
    tunnel: [w325] -> w271
    tunnel: [w324] -> w270
    tunnel: [w331] -> w269
    tunnel: w271 -> [w331]
    tunnel: [w330] -> w268
    tunnel: w270 -> [w330]
    tunnel: w269 -> [w340]
    tunnel: w268 -> [w339]
    tunnel: [w338] -> w28
    tunnel: [w337] -> w76
    frame #0 {
      w318 = FALSE ("Retract Pump 3")
      n156 = local read "Trap 1 (ON/OFF)"() -> (w319:bool)
      n157 = xnode "Read/Write Control"("FPGA VI Reference In"=w327, "error in"=w326, "Direct RF Box  Communication"=FALSE) -> ("FPGA VI Reference Out"=w325:T18, "error out"=w324:errorcluster)
      n158 = local write "Saving..."(FALSE ("Saving Data")) -> ()
      n159 = local write "Stop All"(FALSE ("Stop All")) -> ()
      n160 = local write "Retract Pump 1"(w318) -> ()
      n161 = local write "Retract Pump 3"(w318) -> ()
      n162 = local write "Index"(1.0 ("Index")) -> ()
      n163 = property on="Trap 1 ON" class="Bool (strict)"("Value"=w319) -> ()  [unwired: 2 in, 2 out]
      "Manipulating Trap" <- FALSE ("Manipulating Trap")
    }
    frame #1 {
      n164 = local read "Trap 2 (ON/OFF)"() -> (w329:bool)
      n165 = Wait (ms)(milliseconds to wait=u32 10) -> ()  [unwired: 1 out]
      n166 = property on="Trap 2 ON" class="Bool (strict)"("Val(Sgnl)"=w329) -> ()  [unwired: 2 in, 2 out]
    }
    frame #2 {
      n167 = local read "Scan Range (nm)"() -> (w333:dbl)
      n168 = xnode "Read/Write Control"("FPGA VI Reference In"=w340, "error in"=w339, "FPGA Controls  RF Box"=TRUE ("Direct RF Box  Communication")) -> ("FPGA VI Reference Out"=w338:T18, "error out"=w337:errorcluster)
      n169 = call "Update messages.vi"("Message to add"="UHR-Fleezers ready.", "Old message string"="") -> ("New message string"=w336:string)
      n170 = local write "Messages"(w336) -> ()
      n171 = property on="Scan Range (nm)" class="DigNum (strict)"("Val(Sgnl)"=w333) -> ()  [unwired: 2 in, 2 out]
    }
  }
  n172 = Subtract(x="BD 1 Frequency 1 (MHz)", y="BD 1 Frequency 2 (MHz)") -> (x-y=w190:dbl)
  n173 = Subtract(x="BD 2 Frequency 1 (MHz)", y="BD 2 Frequency 2 (MHz)") -> (x-y=w189:dbl)
  n174 = Square(x=w189) -> (x^2=w187:dbl)
  n175 = Square(x=w190) -> (x^2=w188:dbl)
  n176 = Add(x=w188, y=w187) -> (x+y=w186:dbl)
  n177 = Square Root(x=w186) -> (sqrt(x)=w185:dbl)
  n178 = local write "Trap Delta (MHz)"(w185) -> ()
  n179 = call "IMAQ Create"("Image Name"="APD 1 Image", "Image Type"=w98) -> ("New Image"=w97:T2)  [unwired: 3 in, 1 out]
  n180 = call "IMAQ Create"("Image Name"="APD 2 Image", "Image Type"=w98) -> ("New Image"=w96:T2)  [unwired: 3 in, 1 out]
  n181 = call "IMAQ Create"("Image Name"="Det. X Image", "Image Type"=w98) -> ("New Image"=w95:T2)  [unwired: 3 in, 1 out]
  n182 = call "IMAQ Create"("Image Name"="Det. Y Image", "Image Type"=w98) -> ("New Image"=w94:T2)  [unwired: 3 in, 1 out]
  n183 = Bundle("New Image"=w97, "New Image"=w96, "New Image"=w95, "New Image"=w94) -> (w93:T19)  [unwired: 1 in]
  n184 = call-poly "VISA Configure Serial Port"("VISA resource name"="Bottom  1 Harvard Syringe Pump Serial Port", "baud rate (9600)"=u32 115200, "stop bits (10: 1 bit)"=w34) -> ("VISA resource name out"=w30:refnum<visa-resource-name>, "error out"=w29:errorcluster)  [unwired: 4 in, 7 out]
  n185 = call-poly "VISA Configure Serial Port"("VISA resource name"="Top 3 Harvard Syringe Pump Serial Port", "baud rate (9600)"=u32 115200, "stop bits (10: 1 bit)"=w37) -> ("VISA resource name out"=w32:refnum<visa-resource-name>, "error out"=w31:errorcluster)  [unwired: 4 in, 7 out]
  n186 = call-poly "VISA Configure Serial Port"("VISA resource name"="Sample Chamber Stage Serial Port") -> ("VISA resource name out"=w107:refnum<visa-resource-name>, "error out"=w108:errorcluster)  [unwired: 5 in, 8 out]
  "Stage Control Serial Error" <- w108
  n187 = call-poly "VISA Configure Serial Port"("VISA resource name"="Center Harvard Syringe Pump Serial Port", "baud rate (9600)"=u32 115200, "stop bits (10: 1 bit)"=w91) -> ("VISA resource name out"=w88:refnum<visa-resource-name>, "error out"=w89:errorcluster)  [unwired: 4 in, 7 out]
  n188 = node-c288() -> (w118:T20)  [unwired: 4 out]
  n189 = node-c288() -> (w103:T20)  [unwired: 4 in]
  n190 = disable-structure shown="Disabled" {
    disable-tunnel: [w343 _] -> w249
    disable-tunnel: w28 -> [w342 _]
    frame Disabled {
      n191 = node-c288() -> (w345:T20)  [unwired: 4 out]
      n192 = timed-loop "Rough control of MCL mirror stage (debugging)" {
        tunnel: w342 -> [w348]
        tunnel: [w347] -> w343
        timing: w345 -> [_]
        timing-out: [_] -> w344
        stop <- w347 stop-if-true
        n193 = node-c288() -> ()  [unwired: 2 out]
        n194 = case shown="1" "MCL Mode" {
          tunnel: w348 -> [_ w351 w398]
          frame 0, Default {
          }
          frame 1 {
            n195 = node-c288() -> (w353:T20)  [unwired: 4 out]
            n196 = timed-loop "Oscillate MCL mirror" {
              timing: w353 -> [_]
              timing-out: [_] -> w352
              tunnel: w351 -> [w392]
              i -> [w391]
              stop <- w354 stop-if-true
              n197 = node-c288() -> (w390:i64)  [unwired: 1 out]
              n198 = Multiply(x="AO1", y=32767.0) -> (x*y=w386:dbl)
              n199 = Multiply(x="AO2", y=32767.0) -> (x*y=w381:dbl)
              n200 = Divide(x=w386, y=10.0) -> (x/y=w387:dbl)
              n201 = Divide(x=w381, y=10.0) -> (x/y=w382:dbl)
              n202 = To Word Integer(number=w387) -> (16bit integer=w379:i16)
              n203 = To Word Integer(number=w382) -> (16bit integer=w378:i16)
              n204 = Divide(x=w390, y=i64 1000) -> (x/y=w361:dbl)
              n205 = Multiply(x=w361, y=w391) -> (x*y=w372:dbl)
              n206 = Multiply(x="Osc. freq. (Hz) 2", y=6.283185307179586) -> (x*y=w373:dbl)
              n207 = Multiply(x=w373, y=w372) -> (x*y=w371:dbl)
              n208 = Sine(x=w371) -> (sin(x)=w370:dbl)
              n209 = Multiply(x=w370, y="Osc. amp. (V)") -> (x*y=w368:dbl)
              n210 = Add(x=w368, y="Osc. center (V)") -> (x+y=w366:dbl)
              n211 = Divide(x=w366, y=10.0) -> (x/y=w364:dbl)
              n212 = Multiply(x=w364, y=32767.0) -> (x*y=w359:dbl)
              n213 = Select(t=w359, s="Scan axis", f=w379) -> (s? t:f=w377:dbl)
              n214 = Select(t=w378, s="Scan axis", f=w359) -> (s? t:f=w376:dbl)
              n215 = local read "MCL Mode"() -> (w358:u16)
              n216 = Not Equal?(x=w358, y=u16 1) -> (x != y?=w355:bool)
              n217 = local read "Stop All"() -> (w356:bool)
              n218 = xnode "Read/Write Control"("FPGA VI Reference In"=w392, "AO1"=w377, "AO2"=w376) -> ()  [unwired: 1 in, 2 out]
              n219 = Compound Arithmetic op=OR(w356, w355) -> (w354:bool)
              n220 = node-c288() -> ()  [unwired: 2 out]
            }
            n221 = node-c288(w352) -> ()  [unwired: 1 out]
          }
          frame 2 {
            n222 = case shown="True" "Start Scan" {
              tunnel: w398 -> [_ w410]
              frame False {
              }
              frame True {
                n223 = Subtract(x="End (V)", y="Begin (V)") -> (x-y=w406:dbl)
                n224 = Decrement(x="N Points") -> (x-1=w405:dbl)
                n225 = Divide(x=w406, y=w405) -> (x/y=w403:dbl)
                n226 = for {
                  N: "N Points" -> [_]
                  tunnel: "Begin (V)" -> [w423]
                  tunnel: w410 -> [w415]
                  tunnel: [w414] -> w409 mode=indexing
                  tunnel: w403 -> [w413]
                  tunnel: [w411] -> w402 mode=indexing
                  i -> [w422]
                  n227 = Multiply(x=w413, y=w422) -> (x*y=w421:dbl)
                  n228 = Add(x=w423, y=w421) -> (x+y=w418:dbl)
                  n229 = local read "Scan axis"() -> (w412:bool)
                  n230 = local read "AO1"() -> (w420:dbl)
                  n231 = local read "AO2"() -> (w419:dbl)
                  n232 = Select(t=w418, s=w412, f=w420) -> (s? t:f=w417:dbl)
                  n233 = Select(t=w419, s=w412, f=w418) -> (s? t:f=w416:dbl)
                  n234 = flat-sequence {
                    tunnel: w417 -> [w427]
                    tunnel: w416 -> [w426]
                    tunnel: w415 -> [w424]
                    tunnel: [w437] -> w414
                    tunnel: [w436] -> w411
                    frame #0 {
                      w430 = 10.0 ("y")
                      w425 = 32767.0 ("y")
                      n235 = Multiply(x=w427, y=w425) -> (x*y=w433:dbl)
                      n236 = Multiply(x=w426, y=w425) -> (x*y=w431:dbl)
                      n237 = Divide(x=w433, y=w430) -> (x/y=w434:dbl)
                      n238 = Divide(x=w431, y=w430) -> (x/y=w432:dbl)
                      n239 = To Word Integer(number=w434) -> (16bit integer=w428:i16)
                      n240 = To Word Integer(number=w432) -> (16bit integer=w429:i16)
                      n241 = xnode "Read/Write Control"("FPGA VI Reference In"=w424, "AO1"=w428, "AO2"=w429) -> ()  [unwired: 1 in, 2 out]
                    }
                    frame #1 {
                      n242 = Wait (ms)(milliseconds to wait="DAQ Delay (ms)") -> ()  [unwired: 1 out]
                    }
                    frame #2 {
                      n243 = local read "Slow mean"() -> (w437:dbl)
                      n244 = local read "Sigma"() -> (w436:dbl)
                    }
                  }
                }
                n245 = Bundle("Begin (V)"="Begin (V)", w403, w409) -> (→"MCL Scan":cluster{"Begin (V)":dbl, dbl, dbl[]})  [unwired: 1 out]
                n246 = Bundle("Begin (V)"="Begin (V)", w403, w402) -> (→"MCL Scan 2":cluster{"Begin (V)":dbl, dbl, dbl[]})  [unwired: 1 out]
              }
            }
          }
        }
        n247 = local read "Stop All"() -> (w347:bool)
        n248 = node-c288() -> ()  [unwired: 2 out]
      }
      n249 = node-c288(w344) -> ()  [unwired: 1 out]
    }
    frame Enabled {
    }
  }
  n250 = node-c288(i64 1 ("Period"), 1 ("Processor")) -> (w194:T20)  [unwired: 2 out]
  n251 = node-c288(2 ("Processor")) -> (w116:T20)  [unwired: 3 out]
  n252 = timed-loop "Mouse control: trap position (AOM deflection), set confocal spot from image" {
    tunnel: [w441] -> w201
    tunnel: w28 -> [w440]
    timing: w118 -> [_]
    timing-out: [_] -> w117
    stop <- w441 stop-if-true
    n253 = node-c288() -> ()  [unwired: 2 out]
    n254 = event shown="[0] \"Pane\": Mouse Down" {
      selector: _ -> [_ _]
      dyn-events: _ -> [_ _]
      timeout: _ -> [_ _]
      tunnel: w440 -> [w444 _]
      event Mouse Down {
        n255 = event-data() -> ("Time"=w446:u32, "Coords"=w445:T7, "Button"=w447:u16)  [unwired: 6 out]
        n256 = case shown="1" w447 {
          tunnel: w446 -> [_ _ w553]
          tunnel: w445 -> [_ w484 w551]
          tunnel: w444 -> [_ _ w549]
          frame 0, Default {
          }
          frame 1 {
            n257 = property on="APD 2" class="ImageControl"() -> ("Displayed Image Position"=w454:cluster{"Left":i32, "Top":i32})  [unwired: 2 in, 2 out]
            n258 = property on="APD 1" class="ImageControl"() -> ("Displayed Image Position"=w483:cluster{"Left":i32, "Top":i32})  [unwired: 2 in, 2 out]
            n259 = property on="Detection Laser X" class="ImageControl"() -> ("Displayed Image Position"=w480:cluster{"Left":i32, "Top":i32})  [unwired: 2 in, 2 out]
            n260 = property on="Detection Laser Y" class="ImageControl"() -> ("Displayed Image Position"=w479:cluster{"Left":i32, "Top":i32})  [unwired: 2 in, 2 out]
            n261 = property on="APD 2" class="ImageControl"() -> ("Displayed Image Size"=w453:cluster{"Width":u32, "Height":u32})  [unwired: 2 in, 2 out]
            n262 = property on="APD 1" class="ImageControl"() -> ("Displayed Image Size"=w481:cluster{"Width":u32, "Height":u32})  [unwired: 2 in, 2 out]
            n263 = property on="Detection Laser X" class="ImageControl"() -> ("Displayed Image Size"=w482:cluster{"Width":u32, "Height":u32})  [unwired: 2 in, 2 out]
            n264 = property on="Detection Laser Y" class="ImageControl"() -> ("Displayed Image Size"=w478:cluster{"Width":u32, "Height":u32})  [unwired: 2 in, 2 out]
            n265 = Unbundle By Name(w453) -> ("Width"=w450:u32, "Height"=w449:u32)
            n266 = Unbundle By Name(w454) -> ("Left"=w452:i32, "Top"=w451:i32)
            n267 = Unbundle By Name(w481) -> ("Width"=w475:u32, "Height"=w474:u32)
            n268 = Unbundle By Name(w482) -> ("Width"=w471:u32, "Height"=w470:u32)
            n269 = Unbundle By Name(w478) -> ("Width"=w467:u32, "Height"=w466:u32)
            n270 = Unbundle By Name(w483) -> ("Left"=w477:i32, "Top"=w476:i32)
            n271 = Unbundle By Name(w480) -> ("Left"=w473:i32, "Top"=w472:i32)
            n272 = Unbundle By Name(w479) -> ("Left"=w469:i32, "Top"=w468:i32)
            n273 = Bundle("Left"=w452, "Top"=w451, "Width"=w450, "Height"=w449) -> (w448:T23)  [unwired: 1 in]
            n274 = Bundle("Left"=w477, "Top"=w476, "Width"=w475, "Height"=w474) -> (w465:T23)  [unwired: 1 in]
            n275 = Bundle("Left"=w473, "Top"=w472, "Width"=w471, "Height"=w470) -> (w464:T23)  [unwired: 1 in]
            n276 = Bundle("Left"=w469, "Top"=w468, "Width"=w467, "Height"=w466) -> (w463:T23)  [unwired: 1 in]
            n277 = Build Cluster Array(w448, w465, w464, w463) -> (w462:T24)
            n278 = for {
              tunnel: w484 -> [w495]
              tunnel: w462 -> [w496] mode=indexing
              shift-right: [w493] -> w460
              shift-left: TRUE -> [w494]
              shift-right: [w492] -> w458
              shift-left: _ -> [w488]
              shift-right: [w491] -> w457
              shift-left: _ -> [w487]
              shift-right: [w490] -> w456
              shift-left: _ -> [w486]
              shift-right: [w489] -> w455
              shift-left: _ -> [w485]
              n279 = case shown="True" w494 {
                selector: w494 -> [w501 _]
                tunnel: w496 -> [_ w510]
                tunnel: w495 -> [_ w508]
                tunnel: [w501 w506] -> w493
                tunnel: [w500 w505] -> w492
                tunnel: [w499 w504] -> w491
                tunnel: [w498 w503] -> w490
                tunnel: [w497 w502] -> w489
                tunnel: w488 -> [w500 _]
                tunnel: w487 -> [w499 _]
                tunnel: w486 -> [w498 _]
                tunnel: w485 -> [w497 _]
                frame False {
                }
                frame True {
                  n280 = Unbundle(w510) -> (w509:T23)
                  n281 = call "isclickinwindow.vi"("Image Param"=w509, "Point32"=w508) -> ("4 Y"=w502:i32, "3 Height"=w503:i32, "2 X"=w504:i32, "1 Width"=w505:i32, "In image?"=w507:bool)  [unwired: 1 in]
                  n282 = Not(x=w507) -> (.not. x?=w506:bool)
                }
              }
            }
            n283 = Not(x=w460) -> (.not. x?=w459:bool)
            n284 = case shown="True" w459 {
              tunnel: w457 -> [_ w524]
              tunnel: w455 -> [_ w523]
              tunnel: w458 -> [_ w522]
              tunnel: w456 -> [_ w521]
              frame False {
              }
              frame True {
                w511 = FALSE ("Get Point")
                n285 = local read "Scan lines (y)"() -> (w526:u64)
                n286 = disable-structure shown="Disabled" {
                  frame Disabled {
                  }
                  frame Enabled {
                  }
                }
                n287 = local read "Actual MCL Inc (V)"() -> (w520:dbl)
                n288 = local read "Scan steps (MCL)"() -> (w525:u64)
                n289 = Divide "Y Pix/step"(x=w521, y=w526) -> (x/y=w533:dbl)
                n290 = Divide "Y V/pix"(x=w520, y=w533) -> (x/y=w532:dbl)
